vi "FFScanPositionDefinition.vi"() -> ()   [LabVIEW 2015]
doc: "Use this template to build a user interface event handler design pattern. Use this pattern for dialog boxes and other user interfaces. You also can create and execute user-defined events that the VI can handle the same way as user interface events."
panel:
  out "Array":dbl[](array[numeric])
  in  "OK Button":bool
  in  "Pts":dbl
  in  "dPhi (deg)":dbl
  in  "Start Phi (deg)":dbl
  # "Initial positions"
  # "Delta"
  # "Nbr of points"
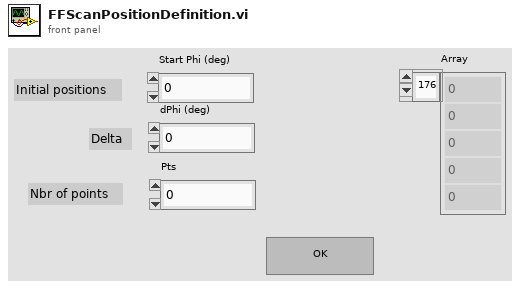
[diagram p1: front panel]
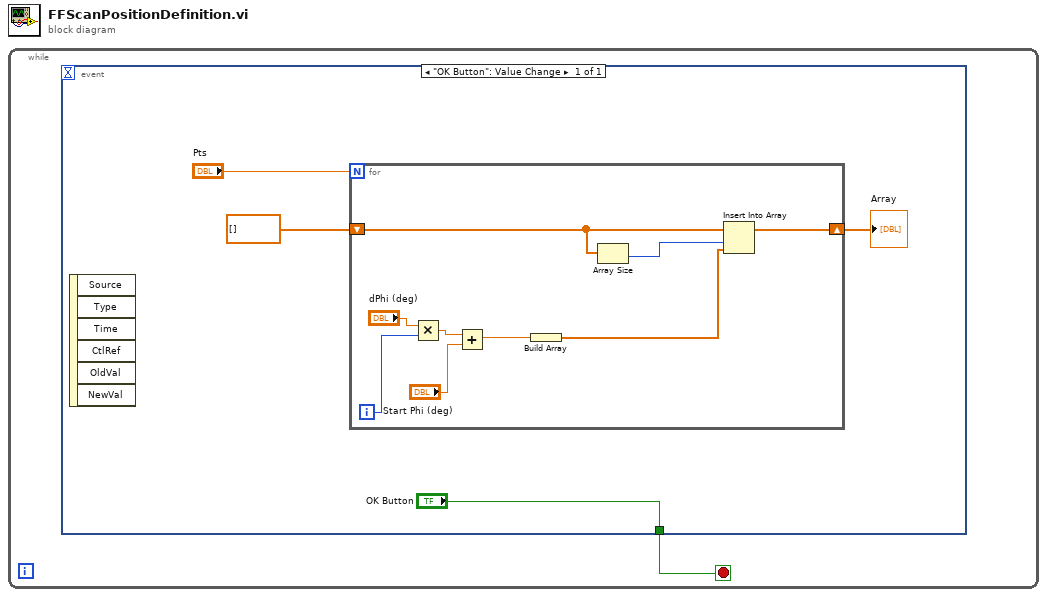
[diagram p0: block diagram]
diagram:
  n1 = while {
    stop <- w1 stop-if-true
    n2 = event shown="[0] \"OK Button\": Value Change" {
      selector: _ -> [_]
      dyn-events: _ -> [_]
      timeout: _ -> [_]
      tunnel: ["OK Button"] -> w1
      event "OK Button": Value Change {
        n3 = event-data() -> ()  [unwired: 1 in, 6 out]
        n4 = for {
          N: "Pts" -> [_]
          shift-right: [w10] -> w2
          shift-left: dbl[] [] -> [w9]
          i -> [w13]
          n5 = Multiply(x="dPhi (deg)", y=w13) -> (x*y=w11:dbl)
          n6 = Add(x=w11, y="Start Phi (deg)") -> (x+y=w8:dbl)
          n7 = Build Array(w8) -> (w7:dbl[])
          n8 = Array Size(array=w9) -> (size(s)=w6:i32)
          n9 = Insert Into Array(array=w9, index=w6, new element=w7) -> (w10:dbl[])
        }
        "Array" <- w2
      }
    }
  }
